vi "CRYConfigure Step Front Panel.vi"(11 "Vi Ref":refnum<vi>) -> ()   [LabVIEW 2013]
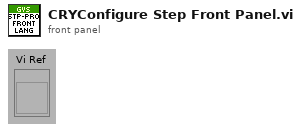
[diagram p1: front panel]
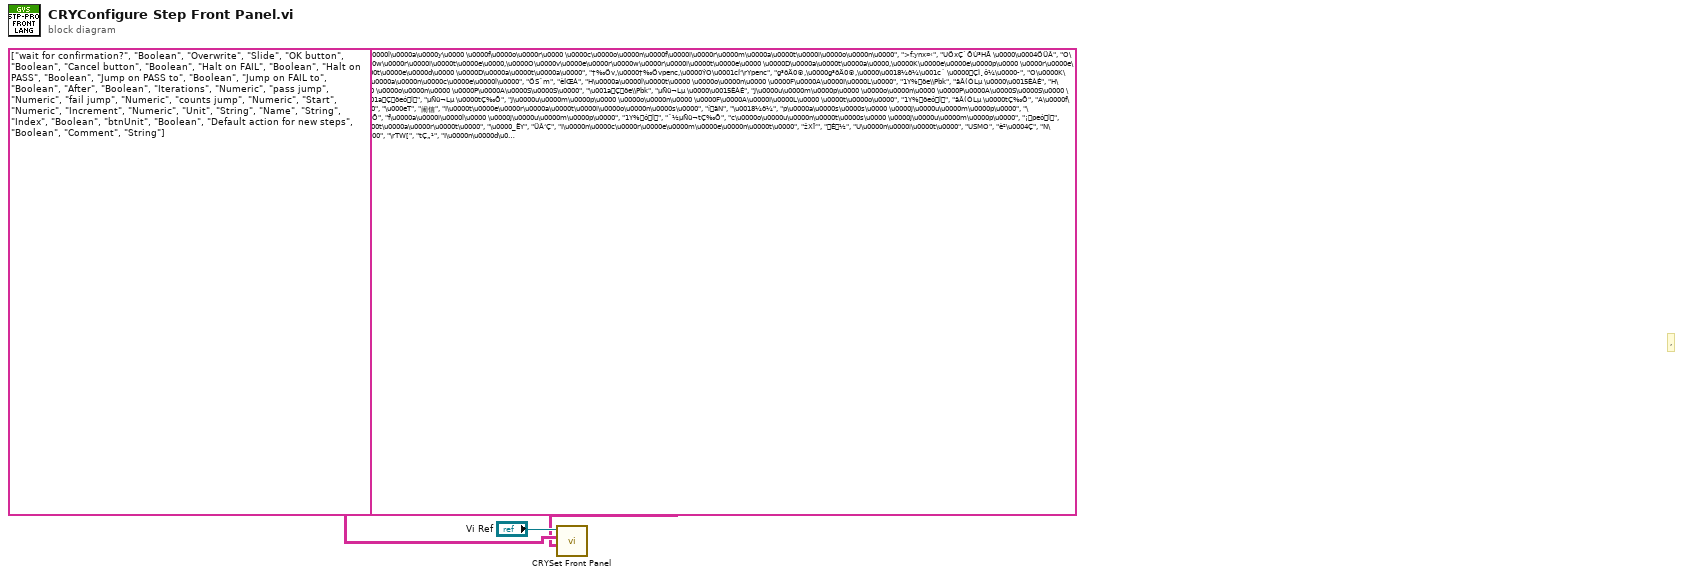
[diagram p0: block diagram]
diagram:
  # ","
  # "Caption, Tab Page, Multilist Header, Button 4"
  # "Control Type"
  # "Control Name and Tab"
  n1 = call "CRYSet Front Panel.vi"("Caption(Boolean Text)"=string[][] [["D\u0000i\u0000s\u0000p\u0000l\u0000a\u0000y\u0000 \u0000f\u0000o\u0000r\u0000 \u0000c\u0000o\u0000n\u0000f\u0000i\u0000r\u0000m\u0000a\u0000t\u0000i\u0000o\u0000n\u0000", ">f:ynx¤‹", "UÖxÇ`ÕÙ³HÅ \u0000\u0004ÖÜÂ"], ["O\u0000v\u0000e\u0000r\u0000w\u0000r\u0000i\u0000t\u0000e\u0000,\u0000O\u0000v\u0000e\u0000r\u0000w\u0000r\u0000i\u0000t\u0000e\u0000 \u0000D\u0000a\u0000t\u0000a\u0000,\u0000K\u0000e\u0000e\u0000p\u0000 \u0000r\u0000e\u0000p\u0000e\u0000a\u0000t\u0000e\u0000d\u0000 \u0000D\u0000a\u0000t\u0000a\u0000", "†‰Öv,\u0000†‰Övpenc,\u0000ÝO\u0001cÍ‘\rYpenc", "g³ðÄ0®,\u0000g³ðÄ0®,\u0000\u0018¼õ¼\u001c´ \u0000ÇÌ¸ô¼\u0000­"], ["O\u0000K\u0000", "nxš[", "UÖxÇ"], ["C\u0000a\u0000n\u0000c\u0000e\u0000l\u0000", "ÖSˆm", "èÍŒÁ"], ["H\u0000a\u0000l\u0000t\u0000 \u0000o\u0000n\u0000 \u0000F\u0000A\u0000I\u0000L\u0000", "1Y%öe\\Pbk", "äÂ(ÓLµ \u0000\u0015ÈÀÉ"], ["H\u0000a\u0000l\u0000t\u0000 \u0000o\u0000n\u0000 \u0000P\u0000A\u0000S\u0000S\u0000", "\u001aÇöe\\Pbk", "µÑü¬Lµ \u0000\u0015ÈÀÉ"], ["J\u0000u\u0000m\u0000p\u0000 \u0000o\u0000n\u0000 \u0000P\u0000A\u0000S\u0000S\u0000 \u0000t\u0000o\u0000", "\u001aÇöeól", "µÑü¬Lµ \u0000tÇ‰Õ"], ["J\u0000u\u0000m\u0000p\u0000 \u0000o\u0000n\u0000 \u0000F\u0000A\u0000I\u0000L\u0000 \u0000t\u0000o\u0000", "1Y%öeól", "äÂ(ÓLµ \u0000tÇ‰Õ"], ["A\u0000f\u0000t\u0000e\u0000r\u0000", "\u000eT", "闹信"], ["I\u0000t\u0000e\u0000r\u0000a\u0000t\u0000i\u0000o\u0000n\u0000s\u0000", "íãN", "\u0018¼õ¼"], ["p\u0000a\u0000s\u0000s\u0000 \u0000j\u0000u\u0000m\u0000p\u0000", "\u001aÇól", "µÑü¬tÇ‰Õ"], ["f\u0000a\u0000i\u0000l\u0000 \u0000j\u0000u\u0000m\u0000p\u0000", "1Y%ól", "ˆ½µÑü¬tÇ‰Õ"], ["c\u0000o\u0000u\u0000n\u0000t\u0000s\u0000 \u0000j\u0000u\u0000m\u0000p\u0000", "¡peól", "tÇ‰ÕÄ¬\u0018Â"], ["S\u0000t\u0000a\u0000r\u0000t\u0000", "\u0000_ËY", "ÜÂ‘Ç"], ["I\u0000n\u0000c\u0000r\u0000e\u0000m\u0000e\u0000n\u0000t\u0000", "žXÏ‘", "É½"], ["U\u0000n\u0000i\u0000t\u0000", "USMO", "è²\u0004Ç"], ["N\u0000a\u0000m\u0000e\u0000", "\rTW[", "tÇ„¹"], ["I\u0000n\u0000d\u0000e\u0000x\u0000", "\u0007cpe", "¨Ì\u0018Â"], ["U\u0000n\u0000i\u0000t\u0000.\u0000.\u0000.\u0000", "USMO.\u0000.\u0000.\u0000", "è²\u0004Ç"], ["D\u0000e\u0000f\u0000a\u0000u\u0000l\u0000t\u0000 \u0000a\u0000c\u0000t\u0000i\u0000o\u0000n\u0000 \u0000f\u0000o\u0000r\u0000 \u0000n\u0000e\u0000w\u0000 \u0000s\u0000t\u0000e\u0000p\u0000s\u0000", "Øž¤‹¨R\\O:N°eek¤š", "0®\u0015ÈÙ³‘Ç$Á\u0015È"], ["C\u0000o\u0000m\u0000m\u0000e\u0000n\u0000t\u0000", "èlã‰", "$Á…º"]], "Control ID and Type(Label Name, Type)"=string[][] [["wait for confirmation?", "Boolean"], ["Overwrite", "Slide"], ["OK button", "Boolean"], ["Cancel button", "Boolean"], ["Halt on FAIL", "Boolean"], ["Halt on PASS", "Boolean"], ["Jump on PASS to", "Boolean"], ["Jump on FAIL to", "Boolean"], ["After", "Boolean"], ["Iterations", "Numeric"], ["pass jump", "Numeric"], ["fail jump", "Numeric"], ["counts jump", "Numeric"], ["Start", "Numeric"], ["Increment", "Numeric"], ["Unit", "String"], ["Name", "String"], ["Index", "Boolean"], ["btnUnit", "Boolean"], ["Default action for new steps", "Boolean"], ["Comment", "String"]], "Vi Ref"="Vi Ref") -> ()  [unwired: 9 in]
